vi "Set_Pin_Status.vi"(6 "Valor pin":string(combo), 8 "error in (no error)":errorcluster, 9 "PIN":i32, 10 "CH":i32, 11 "Cypress in":refnum<class "Cypress.lvclass">) -> (0 "error out":errorcluster, 1 "Expected Response":string, 2 "Command to Send":string, 3 "Cypress out":refnum<class "Cypress.lvclass">)   [LabVIEW 2020, in "Cypress.lvclass"]
doc: "Arma el comando y una presupuestada respuesta para el comando de Set Pin"
uses:
  Cypress.lvclass
  Abstract/Serial Device/Combo Box Comandos.ctl
  Abstract/Serial Device/Combo Box Devices.ctl
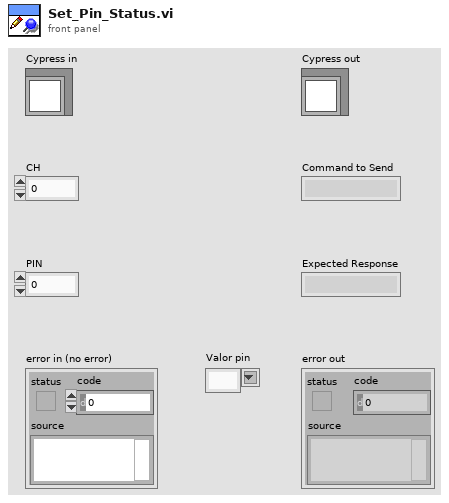
[diagram p1: front panel]
types:
  T1 = typedef "Combo Box Devices.ctl" = string
  T2 = typedef "Combo Box Comandos.ctl" = string
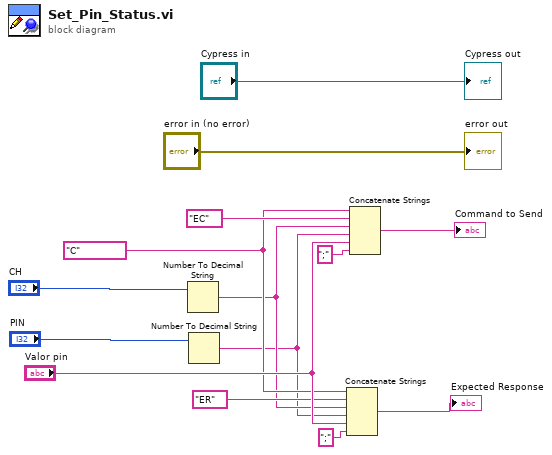
[diagram p0: block diagram]
diagram:
  w8 = T1 "C" ("Serial Devide Brand")
  n1 = Number To Decimal String(number="CH") -> (decimal integer string=w6:string)  [unwired: 1 in]
  n2 = Number To Decimal String(number="PIN") -> (decimal integer string=w3:string)  [unwired: 1 in]
  n3 = Concatenate Strings(w8, T2 "ER" ("Respuesta"), w6, w3, "Valor pin", ";" ("string")) -> (→"Expected Response":string)
  n4 = Concatenate Strings(w8, T2 "EC" ("Command"), w6, w3, "Valor pin", ";" ("string")) -> (→"Command to Send":string)
  "error out" <- "error in (no error)"
  "Cypress out" <- "Cypress in"
